vi "LogDBTimeDep.vi"(0 "Refnum in":T1, 1 "FS-1 [l]":dbl, 2 "FS-2 [l]":dbl, 3 "TS-5 [°C]":dbl, 4 "FS-3 [l]":dbl, 5 "error in (no error)":errorcluster, 6 "db timing":i64, 7 "DS-1 [bar]":dbl, 8 "db":bool, 9 "TS-4 [°C]":dbl, 10 "db Interval [s]":u32, 11 "pHS-1 [pH]":dbl, 12 "Actual Start [f] in":i64) -> (14 "Refnum out":T1, 15 "Actual Start [f] out":i64, 19 "error out":errorcluster)   [LabVIEW 2011]
uses:
  <vilib>/addons/database/Connection.llb/Conn ObjectReference.ctl
  <vilib>/addons/database/NI_Database_API.lvlib
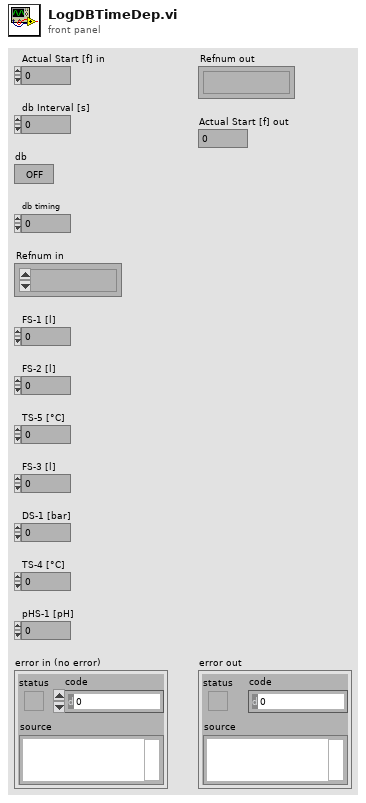
[diagram p1: front panel]
types:
  T1 = typedef "NI_Database_API.lvlib/Conn ObjectReference.ctl" = refnum<k1>
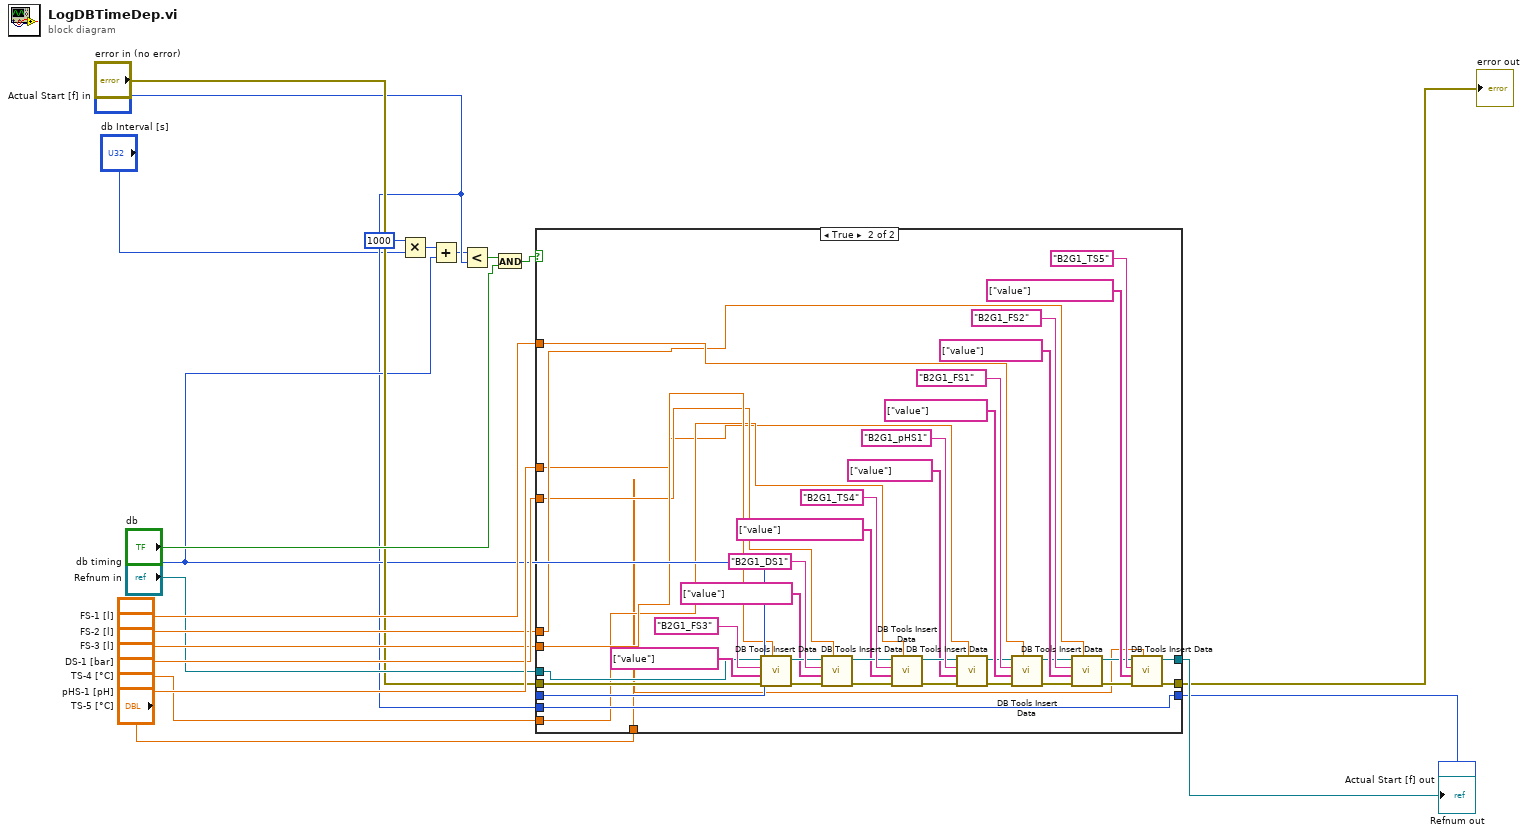
[diagram p0: block diagram]
diagram:
  n1 = Multiply(x=u32 1000, y="db Interval [s]") -> (x*y=w4:u32)
  n2 = Add(x=w4, y="db timing") -> (x+y=w2:i64)
  n3 = Less?(x=w2, y="Actual Start [f] in") -> (x < y?=w3:bool)
  n4 = And(x=w3, y="db") -> (x .and. y?=w14:bool)
  n5 = case shown="True" w14 {
    tunnel: [w24 w32] -> w10
    tunnel: "error in (no error)" -> [w24 w47]
    tunnel: [w23 w48] -> w8
    tunnel: "Actual Start [f] in" -> [_ w48]
    tunnel: "db timing" -> [w23 _]
    tunnel: "Refnum in" -> [w22 w46]
    tunnel: [w22 w33] -> w11
    tunnel: "FS-1 [l]" -> [_ w31]
    tunnel: "FS-2 [l]" -> [_ w30]
    tunnel: "FS-3 [l]" -> [_ w29]
    tunnel: "DS-1 [bar]" -> [_ w28]
    tunnel: "TS-4 [°C]" -> [_ w27]
    tunnel: "pHS-1 [pH]" -> [_ w26]
    tunnel: "TS-5 [°C]" -> [_ w25]
    frame False {
    }
    frame True {
      n6 = call <vilib>:"DB Tools Insert Data.vi"("data"=w29, "error in (no error)"=w47, "columns"=string[] ["value"], "table"="B2G1_FS3", "connection reference"=w46) -> ("error out"=w60:errorcluster, "connection reference out"=w59:T1)  [unwired: 5 in]
      n7 = call <vilib>:"DB Tools Insert Data.vi"("data"=w28, "error in (no error)"=w60, "columns"=string[] ["value"], "table"="B2G1_DS1", "connection reference"=w59) -> ("error out"=w56:errorcluster, "connection reference out"=w57:T1)  [unwired: 5 in]
      n8 = call <vilib>:"DB Tools Insert Data.vi"("data"=w27, "error in (no error)"=w56, "columns"=string[] ["value"], "table"="B2G1_TS4", "connection reference"=w57) -> ("error out"=w53:errorcluster, "connection reference out"=w54:T1)  [unwired: 5 in]
      n9 = call <vilib>:"DB Tools Insert Data.vi"("data"=w26, "error in (no error)"=w53, "columns"=string[] ["value"], "table"="B2G1_pHS1", "connection reference"=w54) -> ("error out"=w43:errorcluster, "connection reference out"=w42:T1)  [unwired: 5 in]
      n10 = call <vilib>:"DB Tools Insert Data.vi"("data"=w31, "error in (no error)"=w43, "columns"=string[] ["value"], "table"="B2G1_FS1", "connection reference"=w42) -> ("error out"=w39:errorcluster, "connection reference out"=w38:T1)  [unwired: 5 in]
      n11 = call <vilib>:"DB Tools Insert Data.vi"("data"=w30, "error in (no error)"=w39, "columns"=string[] ["value"], "table"="B2G1_FS2", "connection reference"=w38) -> ("error out"=w35:errorcluster, "connection reference out"=w34:T1)  [unwired: 5 in]
      n12 = call <vilib>:"DB Tools Insert Data.vi"("data"=w25, "error in (no error)"=w35, "columns"=string[] ["value"], "table"="B2G1_TS5", "connection reference"=w34) -> ("error out"=w32:errorcluster, "connection reference out"=w33:T1)  [unwired: 5 in]
    }
  }
  "Refnum out" <- w11
  "error out" <- w10
  "Actual Start [f] out" <- w8
